vi "ReplaceTypedefByName.vi"(8 "error in (no error)":errorcluster, 9 "Typedef Path":path, 10 "Typedef path name":string="ScriptedCaseStructure", 11 "VI Refnum":refnum<vi>) -> (0 "error out":errorcluster, 3 "VI Refnum":refnum<vi>)   [LabVIEW 2019, in "BlueUtilityScripts.lvlib"]
uses:
  BlueUtilityScripts.lvlib
  <vilib>/Utility/traverseref.llb/TRef TravTarget.ctl
  <vilib>/Utility/error.llb/Error Cluster From Error Code.vi
  <vilib>/ErrorRing/Error Ring.xnode
  <vilib>/Utility/traverseref.llb/VI Scripting - Traverse.lvlib
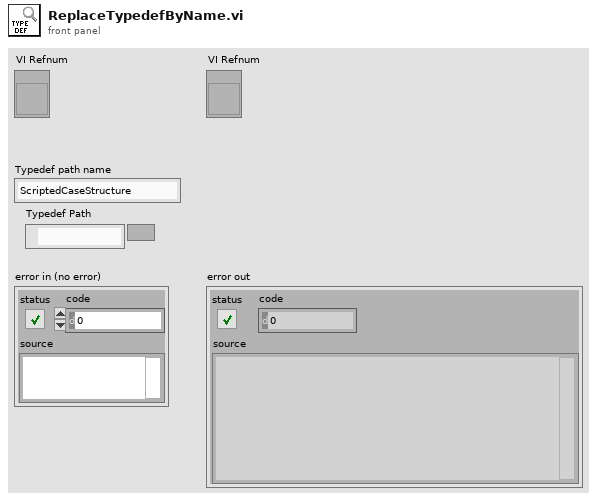
[diagram p1: front panel]
types:
  T1 = typedef "TRef TravTarget.ctl" = enum16{"FP", "BD", "Other"}
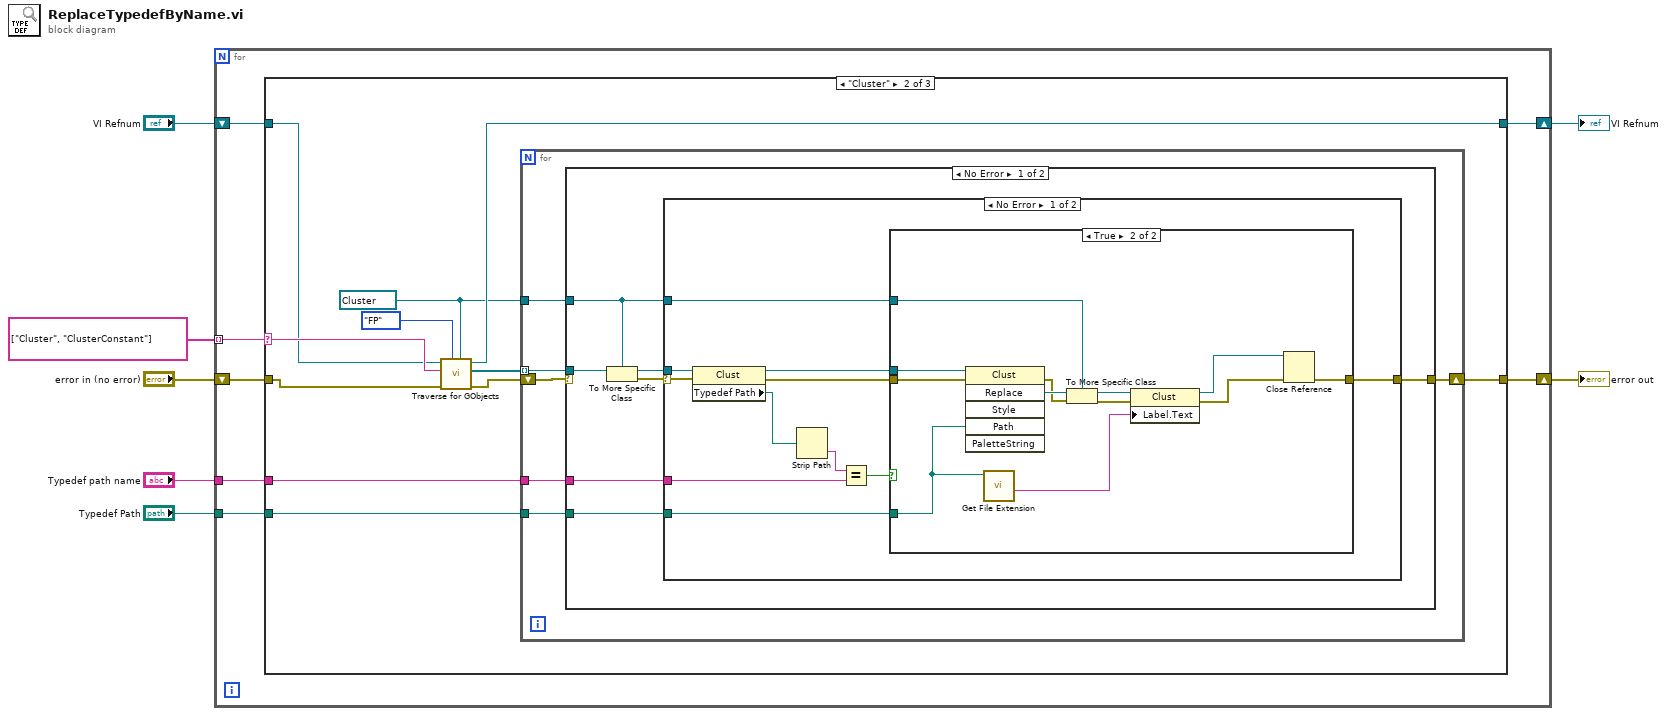
[diagram p0: block diagram]
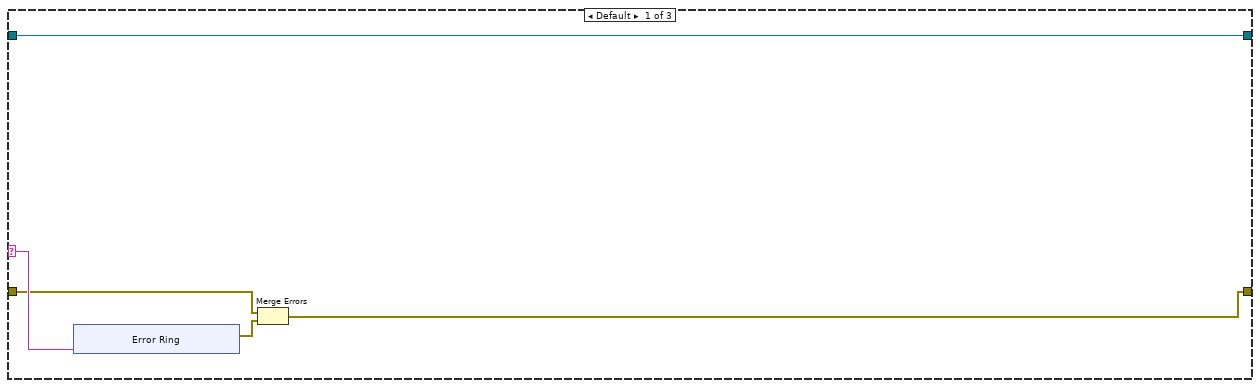
[diagram p2: hidden frame]
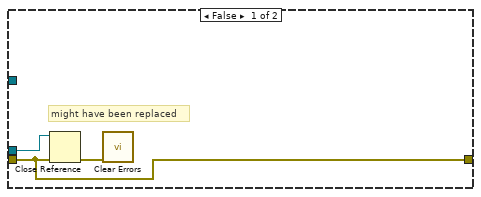
[diagram p3: hidden frame]
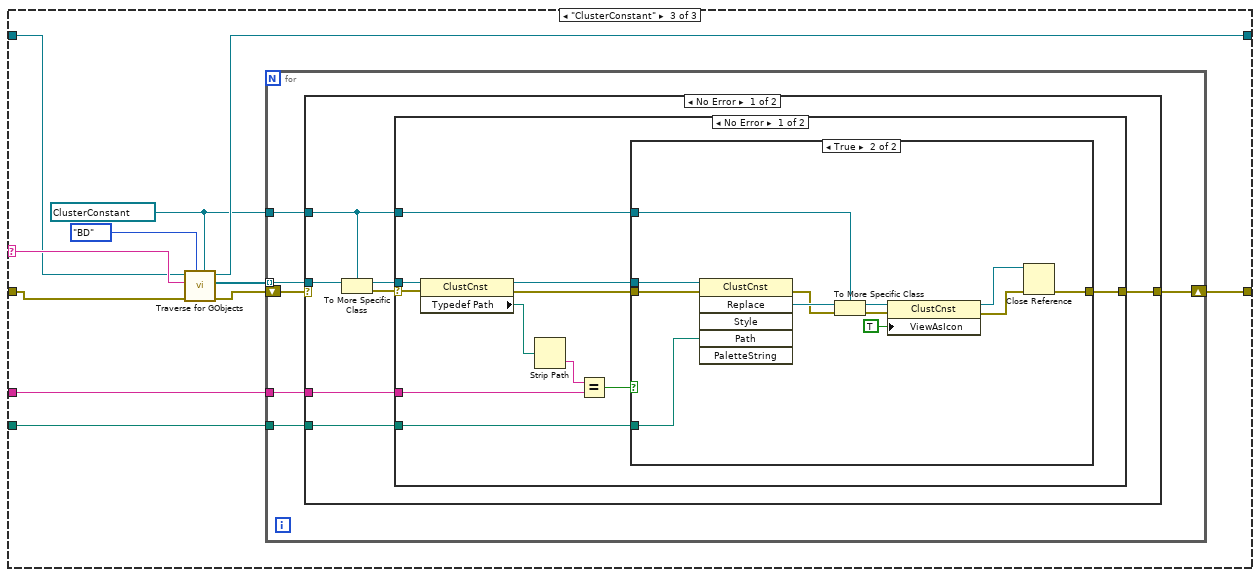
[diagram p6: hidden frame]
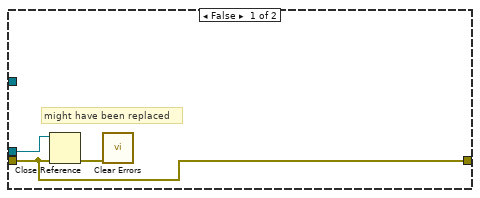
[diagram p7: hidden frame]
diagram:
  n1 = for {
    tunnel: "Typedef path name" -> [w11]
    tunnel: "Typedef Path" -> [w10]
    shift-right: [w12] -> w6
    shift-left: "VI Refnum" -> [w14]
    shift-right: [w9] -> w3
    shift-left: "error in (no error)" -> [w13]
    tunnel: string[] ["Cluster", "ClusterConstant"] -> [w8] mode=indexing
    n2 = case shown="\"Cluster\"" w8 {
      selector: w8 -> [w19 w29 w80]
      tunnel: w14 -> [w15 w28 w79]
      tunnel: w13 -> [w18 w27 w78]
      tunnel: [w15 w36 w87] -> w12
      tunnel: w11 -> [_ w32 w83]
      tunnel: w10 -> [_ w31 w82]
      tunnel: [w16 w30 w81] -> w9
      frame Default {
        n3 = xnode "Error Ring"("parameter 0"=w19) -> ("error out"=w17:errorcluster)
        n4 = Merge Errors(w18, w17) -> (w16:errorcluster)
      }
      frame "Cluster" {
        w34 = refnum<vi> refnum ("Other Refnum")
        n5 = call <vilib>:"Traverse for GObjects.vi"("Other Refnum"=w34, "Traverse Target"=TRef_TravTarget."FP", "error in (no error)"=w27, "Class Name"=w29, "VI Refnum"=w28) -> ("error out"=w33:errorcluster, "References"=w35:refnum<vi>[], "dup VI Refnum"=w36:refnum<vi>)  [unwired: 3 in, 1 out]
        n6 = for {
          tunnel: w35 -> [w43] mode=indexing
          tunnel: w34 -> [w38]
          shift-right: [w39] -> w30
          shift-left: w33 -> [w42]
          tunnel: w32 -> [w41]
          tunnel: w31 -> [w40]
          n7 = case shown="No Error" w42 {
            selector: w42 -> [_ w77]
            tunnel: w43 -> [w48 _]
            tunnel: w41 -> [w47 _]
            tunnel: w40 -> [w46 _]
            tunnel: [w45 w77] -> w39
            tunnel: w38 -> [w44 _]
            frame No Error {
              n8 = To More Specific Class(target class=w44, reference=w48) -> (specific class reference=w49:refnum<vi>, error out=w50:errorcluster)  [unwired: 1 in]
              n9 = case shown="No Error" w50 {
                selector: w50 -> [w61 _]
                tunnel: w49 -> [w60 _]
                tunnel: w47 -> [w58 _]
                tunnel: w46 -> [w56 _]
                tunnel: [w54 _] -> w45
                tunnel: w44 -> [w52 _]
                frame No Error {
                  n10 = property class="Clust"(reference=w60, error in=w61) -> (reference out=w57:refnum<vi>, error out=w55:errorcluster, "Typedef Path"=w53:path)
                  n11 = Strip Path(path=w53) -> (name=w59:string)  [unwired: 1 out]
                  n12 = Equal?(x=w59, y=w58) -> (x = y?=w51:bool)
                  n13 = case shown="True" w51 {
                    tunnel: w57 -> [w64 w76]
                    tunnel: w56 -> [_ w72]
                    tunnel: w55 -> [w62 w75]
                    tunnel: [w62 w74] -> w54
                    tunnel: w52 -> [_ w73]
                    frame False {
                      # "might have been replaced"
                      n14 = Close Reference(reference=w64, error in (no error)=w62) -> (error out=w63:errorcluster)
                      n15 = call <vilib>:"Clear Errors.vi"("error in (no error)"=w63) -> ()  [unwired: 5 in, 2 out]
                    }
                    frame True {
                      n16 = invoke class="Clust" method="Replace"(reference=w76, error in=w75, "Path"=w72) -> (error out=w70:errorcluster, "Replace"=w71:refnum<vi>)  [unwired: 3 in, 4 out]
                      n17 = call <vilib>:"Get File Extension.vi"("file"=w72) -> ("filename without extension"=w68:string)  [unwired: 6 in, 4 out]
                      n18 = To More Specific Class(target class=w73, reference=w71, error in=w70) -> (specific class reference=w69:refnum<vi>, error out=w67:errorcluster)
                      n19 = property class="Clust"(reference=w69, error in=w67, "Label.Text"=w68) -> (reference out=w66:refnum<vi>, error out=w65:errorcluster)
                      n20 = Close Reference(reference=w66, error in (no error)=w65) -> (error out=w74:errorcluster)
                    }
                  }
                }
                frame Error {
                  # "no longer exists"
                }
              }
            }
            frame Error {
            }
          }
        }
      }
      frame "ClusterConstant" {
        w85 = refnum<vi> refnum ("Other Refnum")
        n21 = call <vilib>:"Traverse for GObjects.vi"("Other Refnum"=w85, "Traverse Target"=TRef_TravTarget."BD", "error in (no error)"=w78, "Class Name"=w80, "VI Refnum"=w79) -> ("error out"=w84:errorcluster, "References"=w86:refnum<vi>[], "dup VI Refnum"=w87:refnum<vi>)  [unwired: 3 in, 1 out]
        n22 = for {
          tunnel: w86 -> [w94] mode=indexing
          tunnel: w85 -> [w89]
          shift-right: [w90] -> w81
          shift-left: w84 -> [w93]
          tunnel: w83 -> [w92]
          tunnel: w82 -> [w91]
          n23 = case shown="No Error" w93 {
            selector: w93 -> [_ w128]
            tunnel: w94 -> [w99 _]
            tunnel: w92 -> [w98 _]
            tunnel: w91 -> [w97 _]
            tunnel: [w96 w128] -> w90
            tunnel: w89 -> [w95 _]
            frame No Error {
              n24 = To More Specific Class(target class=w95, reference=w99) -> (specific class reference=w100:refnum<vi>, error out=w101:errorcluster)  [unwired: 1 in]
              n25 = case shown="No Error" w101 {
                selector: w101 -> [w112 _]
                tunnel: w100 -> [w111 _]
                tunnel: w98 -> [w109 _]
                tunnel: w97 -> [w107 _]
                tunnel: [w105 _] -> w96
                tunnel: w95 -> [w103 _]
                frame No Error {
                  n26 = property class="ClustCnst"(reference=w111, error in=w112) -> (reference out=w108:refnum<vi>, error out=w106:errorcluster, "Typedef Path"=w104:path)
                  n27 = Strip Path(path=w104) -> (name=w110:string)  [unwired: 1 out]
                  n28 = Equal?(x=w110, y=w109) -> (x = y?=w102:bool)
                  n29 = case shown="True" w102 {
                    tunnel: w108 -> [w115 w127]
                    tunnel: w107 -> [_ w126]
                    tunnel: w106 -> [w113 w125]
                    tunnel: [w113 w124] -> w105
                    tunnel: w103 -> [_ w123]
                    frame False {
                      # "might have been replaced"
                      n30 = Close Reference(reference=w115, error in (no error)=w113) -> (error out=w114:errorcluster)
                      n31 = call <vilib>:"Clear Errors.vi"("error in (no error)"=w114) -> ()  [unwired: 5 in, 2 out]
                    }
                    frame True {
                      n32 = invoke class="ClustCnst" method="Replace"(reference=w127, error in=w125, "Path"=w126) -> (error out=w121:errorcluster, "Replace"=w122:refnum<vi>)  [unwired: 3 in, 4 out]
                      n33 = To More Specific Class(target class=w123, reference=w122, error in=w121) -> (specific class reference=w120:refnum<vi>, error out=w118:errorcluster)
                      n34 = property class="ClustCnst"(reference=w120, error in=w118, "ViewAsIcon"=TRUE ("View As Icon")) -> (reference out=w117:refnum<vi>, error out=w116:errorcluster)
                      n35 = Close Reference(reference=w117, error in (no error)=w116) -> (error out=w124:errorcluster)
                    }
                  }
                }
                frame Error {
                  # "was deleted"
                }
              }
            }
            frame Error {
            }
          }
        }
      }
    }
  }
  "VI Refnum" <- w6
  "error out" <- w3
